vi "PanelWizard_UpdateDisplay.vi"(9 "Container State":T1, 10 "Display State In":T2={"DisplayStyle"=enum."3D Style", "LaunchType"=enum."LaunchHDV", "UserVIPath"=path "", "Button Text"="", "UseDefaultButtonText?"=FALSE, "Run User VI?"=TRUE, "CommandLine"="", "StandardInput"="", "Working Directory"=path ""} caption="State", 11 "Button Refs":refnum<vi>[](array[refnum])) -> ()   [LabVIEW 2012, in "PanelWizard.xctl"]
uses:
  PanelWizard.xctl
  PanelWizard_State.ctl
  PanelWizard_DisplayType.ctl
  PanelWizard_LaunchOptions.ctl
  <vilib>/_xctls/Container State.ctl
  <vilib>/_xctls/XControlSupport.lvlib
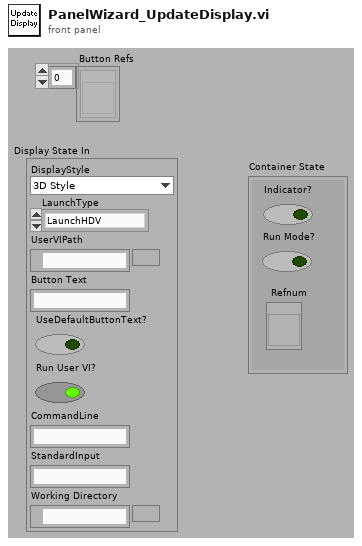
[diagram p1: front panel]
types:
  T1 = typedef "XControlSupport.lvlib/Container State.ctl" = cluster{"Indicator?":bool, "Run Mode?":bool, " Refnum":refnum<vi>}
  T2 = typedef "PanelWizard.xctl/PanelWizard_State.ctl" = cluster{"DisplayStyle":T3, "LaunchType":T4, "UserVIPath":path, "Button Text":string, "UseDefaultButtonText?":bool, "Run User VI?":bool, "CommandLine":string, "StandardInput":string, "Working Directory":path}
  T3 = typedef "PanelWizard.xctl/PanelWizard_DisplayType.ctl" = enum16{"3D Style", "LabVIEW Classic Style", "System Style"}
  T4 = typedef "PanelWizard.xctl/PanelWizard_LaunchOptions.ctl" = enum16{"LaunchHDV", "LaunchSVMonitor", "LaunchUserVI", "Run command line"}
  T5 = typedef "LVBoundsTypeDef.ctl" = cluster{"Width":u32, "Height":u32}
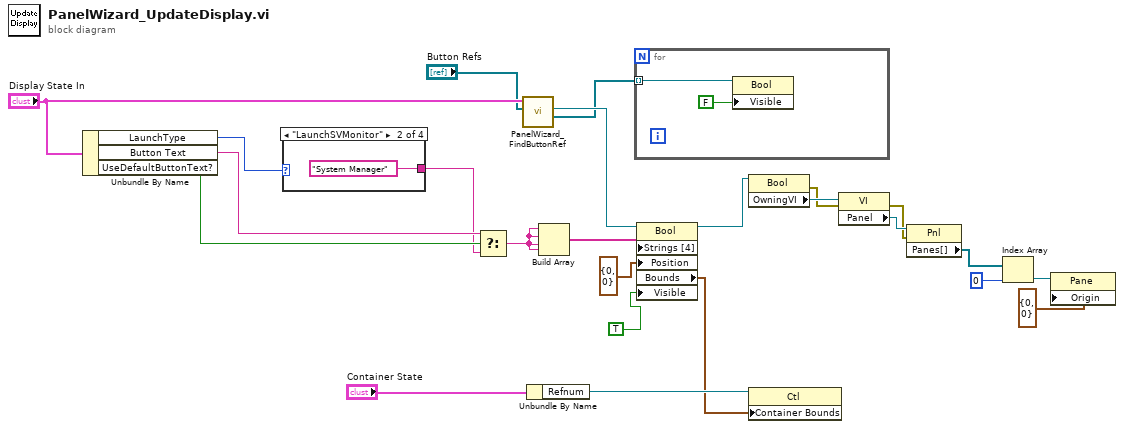
[diagram p0: block diagram]
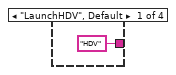
[diagram p2: hidden frame]
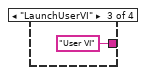
[diagram p3: hidden frame]
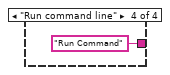
[diagram p4: hidden frame]
diagram:
  n1 = Unbundle By Name("Display State In") -> ("LaunchType"=w19:T4, "Button Text"=w24:string, "UseDefaultButtonText?"=w23:bool)
  n2 = case shown="\"LaunchSVMonitor\"" w19 {
    tunnel: ["HDV" ("Button Text") "System Manager" ("Button Text") "User VI" ("Button Text") "Run Command" ("Button Text")] -> w21
    frame "LaunchHDV", Default {
    }
    frame "LaunchSVMonitor" {
    }
    frame "LaunchUserVI" {
    }
    frame "Run command line" {
    }
  }
  n3 = Select(t=w24, s=w23, f=w21) -> (s? t:f=w22:string)
  n4 = call "PanelWizard_FindButtonRef.vi"("ButtonRefs"="Button Refs", "Display State In"="Display State In") -> ("Disabled Buttons [ref]"=w1:refnum<vi>[], "Enabled Button (ref)"=w3:refnum<vi>)  [unwired: 6 in, 2 out]
  n5 = Unbundle By Name("Container State") -> ("Refnum"=w7:refnum<vi>)
  n6 = Build Array(w22, w22, w22, w22) -> (w20:string[])
  n7 = for {
    tunnel: w1 -> [w29] mode=indexing
    n8 = property on="Property Node" class="Bool"(reference=w29, "Visible"=FALSE) -> ()  [unwired: 1 in, 2 out]
  }
  n9 = property on="Property Node" class="Bool"(reference=w3, "Strings [4]"=w20, "Position"=cluster{"Left":i32, "Top":i32} {"Left"=0, "Top"=0}, "Visible"=TRUE) -> (reference out=w17:refnum<vi>, "Bounds"=w6:T5)  [unwired: 1 in, 1 out]
  n10 = property class="Bool"(reference=w17) -> (error out=w15:errorcluster, "OwningVI"=w16:refnum<vi>)  [unwired: 1 in, 1 out]
  n11 = property class="Ctl"(reference=w7, "Container Bounds"=w6) -> ()  [unwired: 1 in, 2 out]
  n12 = property class="VI"(reference=w16, error in=w15) -> (error out=w13:errorcluster, "Panel"=w14:refnum<vi>)  [unwired: 1 out]
  n13 = property class="Pnl"(reference=w14, error in=w13) -> ("Panes[]"=w12:refnum<vi>[])  [unwired: 2 out]
  n14 = Index Array(array=w12, index=0) -> (element=w10:refnum<vi>)
  n15 = property class="Pane"(reference=w10, "Origin"=cluster{"Horizontal":i16, "Vertical":i16} {"Horizontal"=0, "Vertical"=0}) -> ()  [unwired: 1 in, 2 out]
